vi "Horizontal Panel (2).vi"() -> ()   [LabVIEW 2013, in "PanelDataNode.lvclass"]
uses:
  PanelDataNode.lvclass
  PanelObject/PanelObject.lvclass
  Split Mode.ctl
  PanelLinkNode/PanelLinkNode.lvclass
panel:
  in  "Node*":refnum<data-value>
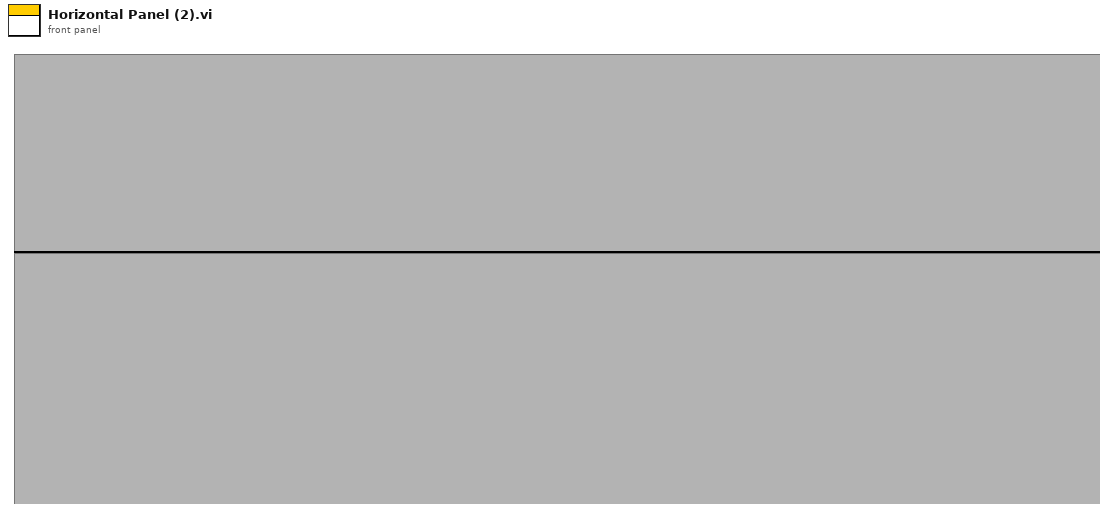
[diagram p1: front panel]
types:
  T1 = typedef "PanelDataNode.lvclass/Split Mode.ctl" = enum16{"Horizontal(up)", "Vertical(left)", "Horizontal(down)", "Vertical(right)"}
  T2 = cluster{"ChildNode*":refnum<data-value>, "Split Mode":T1}
  T3 = cluster{"ChildNode*":refnum<data-value>, "VI*":refnum<vi>}
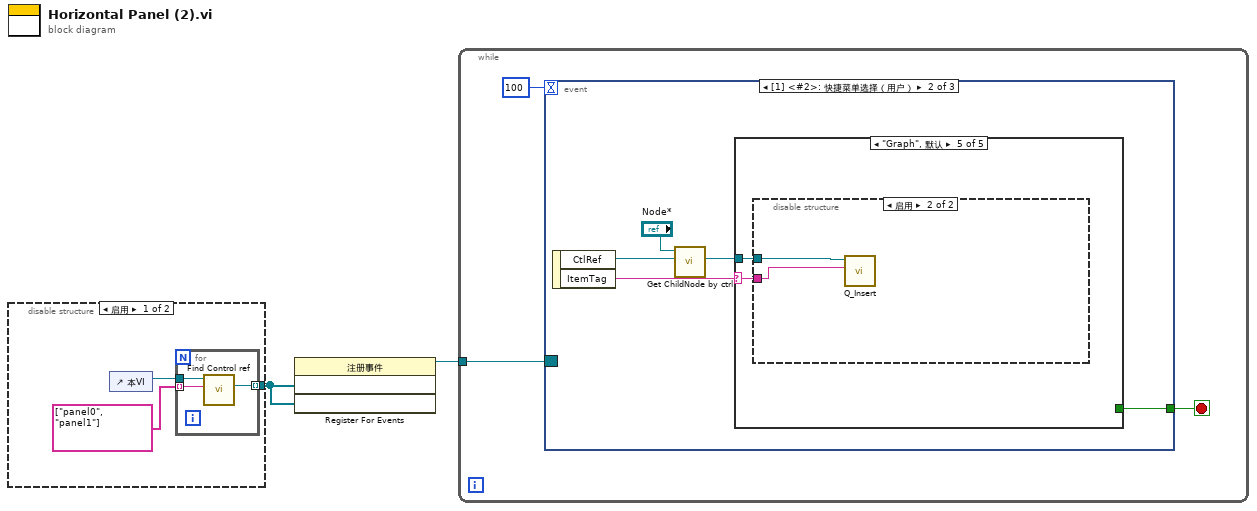
[diagram p0: block diagram]
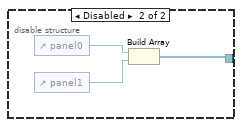
[diagram p2: hidden frame]
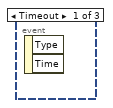
[diagram p3: hidden frame]
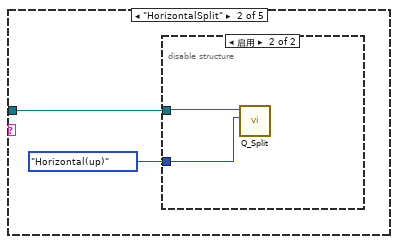
[diagram p5: hidden frame]
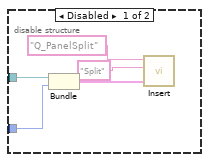
[diagram p6: hidden frame]
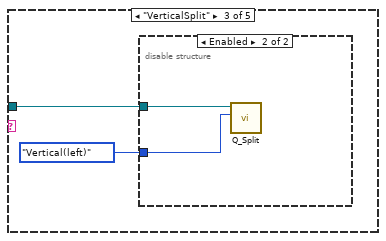
[diagram p7: hidden frame]
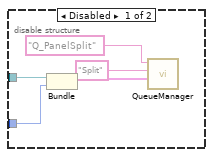
[diagram p8: hidden frame]
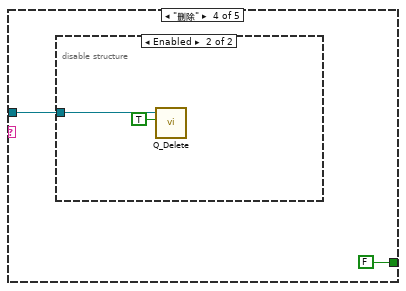
[diagram p9: hidden frame]
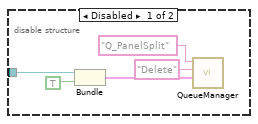
[diagram p10: hidden frame]
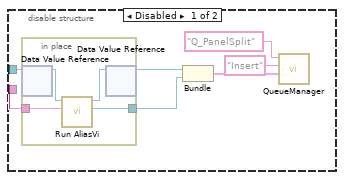
[diagram p11: hidden frame]
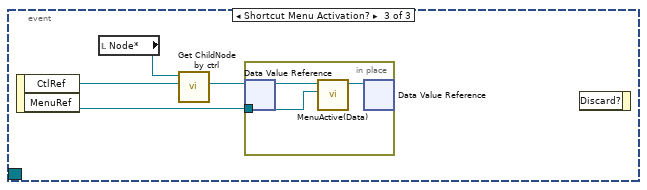
[diagram p12: hidden frame]
diagram:
  n1 = disable-structure shown="启用" {
    disable-tunnel: [w3 w9] -> w1
    frame Enabled {
      n2 = control-ref of="本VI"() -> (w5:refnum<vi>)
      n3 = for {
        tunnel: w5 -> [w8]
        tunnel: string[] ["panel0", "panel1"] -> [w7] mode=indexing
        tunnel: [w6] -> w3 mode=indexing
        n4 = call "Find Control ref.vi"("control name"=w7, "panelvi*"=w8) -> ("ctrl*"=w6:refnum<vi>)  [unwired: 7 in, 2 out]
      }
    }
    frame Disabled {
      n5 = control-ref of="panel0"() -> (w11:refnum<vi>)
      n6 = control-ref of="panel1"() -> (w10:refnum<vi>)
      n7 = Build Array(w11, w10) -> (w9:refnum<vi>[])
    }
  }
  n8 = register-events(w1, w1) -> (reference out=w2:refnum<event-registration>)  [unwired: 2 in, 1 out]
  n9 = while {
    tunnel: w2 -> [w13]
    stop <- w12 stop-if-true
    n10 = event shown="[1] <#2>: 快捷菜单选择（用户）" {
      selector: w13 -> [_ _ _]
      dyn-events: _ -> [_ _ _]
      timeout: 100 -> [_ _ _]
      tunnel: [_ w15 _] -> w12
      event Timeout {
        n11 = event-data() -> ()  [unwired: 1 in, 2 out]
      }
      event Shortcut Menu Selection (User) {
        n12 = event-data() -> ("CtlRef"=w19:refnum<vi>, "ItemTag"=w16:string)  [unwired: 1 in]
        n13 = call "Get ChildNode by ctrl.vi"("ctr*"=w19, "Node*"="Node*") -> ("ChildNode*"=w17:refnum<data-value>)  [unwired: 8 in, 1 out]
        n14 = case shown="\"Graph\", 默认" w16 {
          selector: w16 -> [_ _ _ _ w48]
          tunnel: w17 -> [_ w21 w29 w38 w47]
          tunnel: [_ _ _ FALSE _] -> w15
          frame "假" {
          }
          frame "HorizontalSplit" {
            n15 = disable-structure shown="启用" {
              disable-tunnel: w21 -> [w26 w28]
              disable-tunnel: Split_Mode."Horizontal(up)" ("Split Mode") -> [w25 w27]
              frame Disabled {
                n16 = Bundle("ChildNode*"=w26, "Split Mode"=w25) -> (w24:T2)  [unwired: 1 in]
                n17 = call "Insert.vi"("Data"=w24, "Event"="Split", "QueueName"="Q_PanelSplit") -> ()  [unwired: 7 in, 2 out]
              }
              frame Enabled {
                n18 = call "Q_Split.vi"("Split Mode"=w27, "ChildNode*"=w28) -> ()  [unwired: 9 in, 1 out]
              }
            }
          }
          frame "VerticalSplit" {
            n19 = disable-structure shown="Enabled" {
              disable-tunnel: Split_Mode."Vertical(left)" ("Split Mode") -> [w35 w37]
              disable-tunnel: w29 -> [w34 w36]
              frame Disabled {
                n20 = Bundle("ChildNode*"=w34, "Split Mode"=w35) -> (w31:T2)  [unwired: 1 in]
                n21 = call-poly "QueueManager.vi"("Data"=w31, "Event"="Split", "QueueName"="Q_PanelSplit") -> ()  [unwired: 7 in, 2 out]
              }
              frame Enabled {
                n22 = call "Q_Split.vi"("Split Mode"=w37, "ChildNode*"=w36) -> ()  [unwired: 9 in, 1 out]
              }
            }
          }
          frame "删除" {
            n23 = disable-structure shown="Enabled" {
              disable-tunnel: w38 -> [w44 w46]
              frame Disabled {
                n24 = Bundle("ChildNode*"=w44, TRUE) -> (w43:cluster{"ChildNode*":refnum<data-value>, bool})  [unwired: 1 in]
                n25 = call-poly "QueueManager.vi"("Data"=w43, "Event"="Delete", "QueueName"="Q_PanelSplit") -> ()  [unwired: 7 in, 2 out]
              }
              frame Enabled {
                n26 = call "Q_Delete.vi"("CloseVI?(T)"=TRUE, "ChildNode*"=w46) -> ()  [unwired: 9 in, 1 out]
              }
            }
          }
          frame "Graph", Default {
            n27 = disable-structure shown="启用" {
              disable-tunnel: w48 -> [w52 w60]
              disable-tunnel: w47 -> [w51 w61]
              frame Disabled {
                n28 = in-place {
                  in-place-border: w52 -> [w59]
                  in-place-border: [w56] -> w49
                  n29 = in-place-dvr #1(w51) -> (w58:refnum<class "PanelDataNode.lvclass">)  [unwired: 1 out]
                  n30 = call-dynamic "Run AliasVi.vi"("Vi Alias"=w59, "PanelDataNode 输入"=w58) -> ("VI*"=w56:refnum<vi>, "PanelDataNode 输出"=w57:refnum<class "PanelDataNode.lvclass">)  [unwired: 7 in, 1 out]
                  n31 = in-place-dvr #1(w57) -> (w50:refnum<data-value>)  [unwired: 1 out]
                }
                n32 = Bundle("ChildNode*"=w50, "VI*"=w49) -> (w55:T3)  [unwired: 1 in]
                n33 = call-poly "QueueManager.vi"("Data"=w55, "Event"="Insert", "QueueName"="Q_PanelSplit") -> ()  [unwired: 7 in, 2 out]
              }
              frame Enabled {
                n34 = call "Q_Insert.vi"("Vi Alias"=w60, "ChildNode*"=w61) -> ()  [unwired: 9 in, 1 out]
              }
            }
          }
        }
      }
      event Shortcut Menu Activation? {
        n35 = event-data() -> ("CtlRef"=w65:refnum<vi>, "MenuRef"=w62:refnum<k9>)  [unwired: 1 in]
        n36 = local read "Node*"() -> (w64:refnum<data-value>)
        n37 = call "Get ChildNode by ctrl.vi"("ctr*"=w65, "Node*"=w64) -> ("ChildNode*"=w63:refnum<data-value>)  [unwired: 8 in, 1 out]
        n38 = in-place {
          in-place-border: w62 -> [w67]
          n39 = in-place-dvr #2(w63) -> (w68:refnum<class "PanelDataNode.lvclass">)  [unwired: 1 out]
          n40 = call-dynamic "MenuActive(Data).vi"("菜单引用"=w67, "PanelDataNode 输入"=w68) -> ("PanelDataNode 输出"=w66:refnum<class "PanelDataNode.lvclass">)  [unwired: 7 in, 2 out]
          n41 = in-place-dvr #2(w66) -> ()  [unwired: 2 out]
        }
        n42 = event-data() -> ()  [unwired: 2 in, 1 out]
      }
    }
  }
